vi "TMC_Merge_Cluster.vi"(0 "TMC-Status":T1, 1 "TMC-Control":T2) -> (3 "TMC Cluster":T3)   [LabVIEW 2019]
uses:
  Torque_TMC/TMCCluster.ctl
  Torque_TMC/TMC_Control.ctl
  Torque_TMC/TMC_Status.ctl
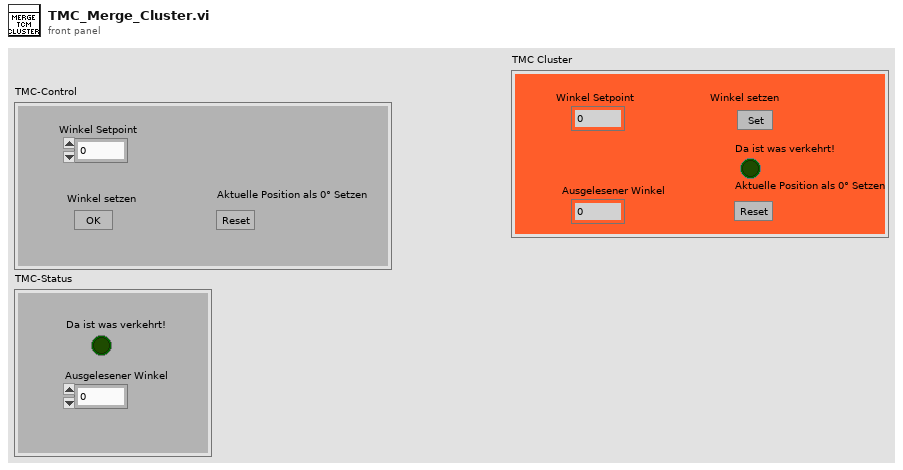
[diagram p1: front panel]
types:
  T1 = typedef "TMC_Status.ctl" = cluster{"Ausgelesener Winkel":dbl, "Da ist was verkehrt!":bool}
  T2 = typedef "TMC_Control.ctl" = cluster{"Winkel Setpoint":dbl, "Aktuelle Position als 0° Setzen":bool, "Winkel setzen":bool}
  T3 = typedef "TMCCluster.ctl" = cluster{"Winkel Setpoint":dbl, "Ausgelesener Winkel":dbl, "Aktuelle Position als 0° Setzen":bool, "Da ist was verkehrt!":bool, "Winkel setzen":bool}
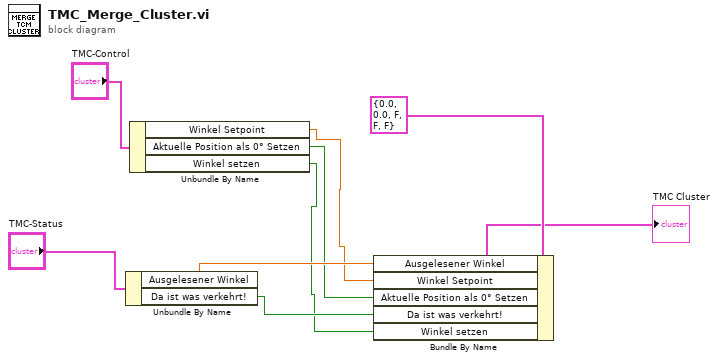
[diagram p0: block diagram]
diagram:
  n1 = Unbundle By Name("TMC-Status") -> ("Ausgelesener Winkel"=w4:dbl, "Da ist was verkehrt!"=w5:bool)
  n2 = Unbundle By Name("TMC-Control") -> ("Winkel Setpoint"=w1:dbl, "Aktuelle Position als 0° Setzen"=w3:bool, "Winkel setzen"=w2:bool)
  n3 = Bundle By Name(cluster=T3 {"Winkel Setpoint"=0.0, "Ausgelesener Winkel"=0.0, "Aktuelle Position als 0° Setzen"=FALSE, "Da ist was verkehrt!"=FALSE, "Winkel setzen"=FALSE} ("TMC Cluster 2"), "Ausgelesener Winkel"=w4, "Winkel Setpoint"=w1, "Aktuelle Position als 0° Setzen"=w3, "Da ist was verkehrt!"=w5, "Winkel setzen"=w2) -> (→"TMC Cluster":T3)
